vi "VCO-sctl-3.vi"(6 "Ready For Output":bool, 8 "Input Valid":bool, 10 "param":T1={"base freq (Hz)"=[20123.0, 20123.0, 20123.0], "P gain"=[1234.0, 1234.0, 1234.0], "I gain"=[1.0, 1.0, 1.0], "LP1 coeffs"=[-1025014616, 2098093632, 165702, -1053286467, 2126356551, 167935, -1025014616, 2098093632, 165702, -1053286467, 2126356551, 167935, -1025014616, 2098093632, 165702, -1053286467, 2126356551, 167935], "scope on"=FALSE, "scope channel"=0, "scope signal"=0, "notch coeff"=[-1025014616, 2098093632, 165702, -1053286467, 2126356551, 167935, -1025014616, 2098093632, 165702]}, 11 "freq error":fxp<+/-,21,11>) -> (0 "Output Valid":bool, 3 "phase":fxp<+,26,1>, 4 "Ready For Input":bool=TRUE)   [LabVIEW 2018, in "SCTL.lvlib"]
doc: "This VI is used in four wire handshake."
uses:
  SCTL.lvlib
  param-sctl-pll.ctl
  <vilib>/rvi/FXPMathLib/FxpAdd/XNode/nifxpmath_Add.xnode
  <vilib>/rvi/FXPMathLib/FxpMul/XNode/nifxpmath_Multiplier.xnode
  <vilib>/rvi/FXPMathLib/sim/FxpSim.dll
panel:
  # "Inputs"
  # "Outputs"
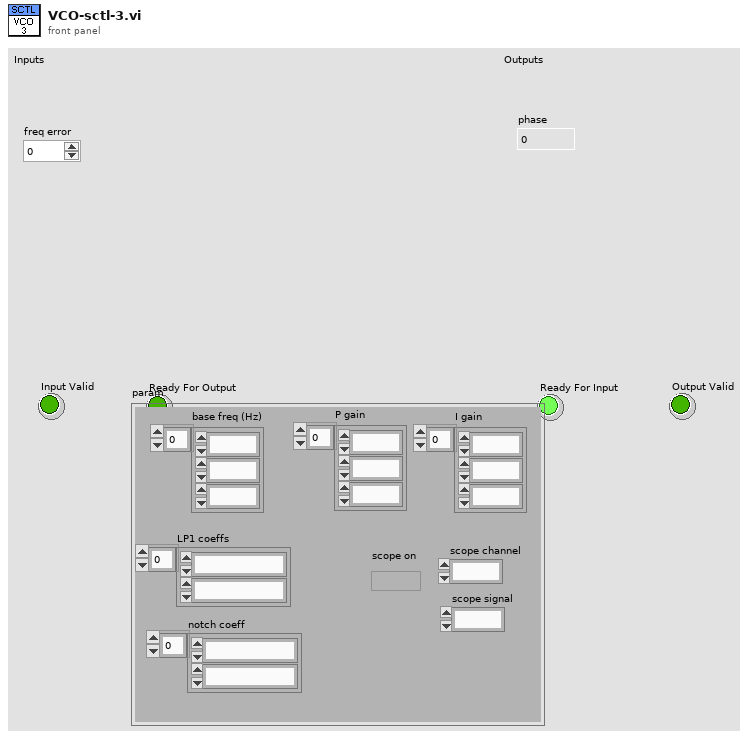
[diagram p1: front panel]
types:
  T1 = typedef "SCTL.lvlib/param-sctl-pll.ctl" = cluster{"base freq (Hz)":fxp<+,17,17>[], "P gain":fxp<+,14,14>[], "I gain":fxp<+,20,6>[], "LP1 coeffs":i32[], "scope on":bool, "scope channel":u8, "scope signal":u8, "notch coeff":i32[]}
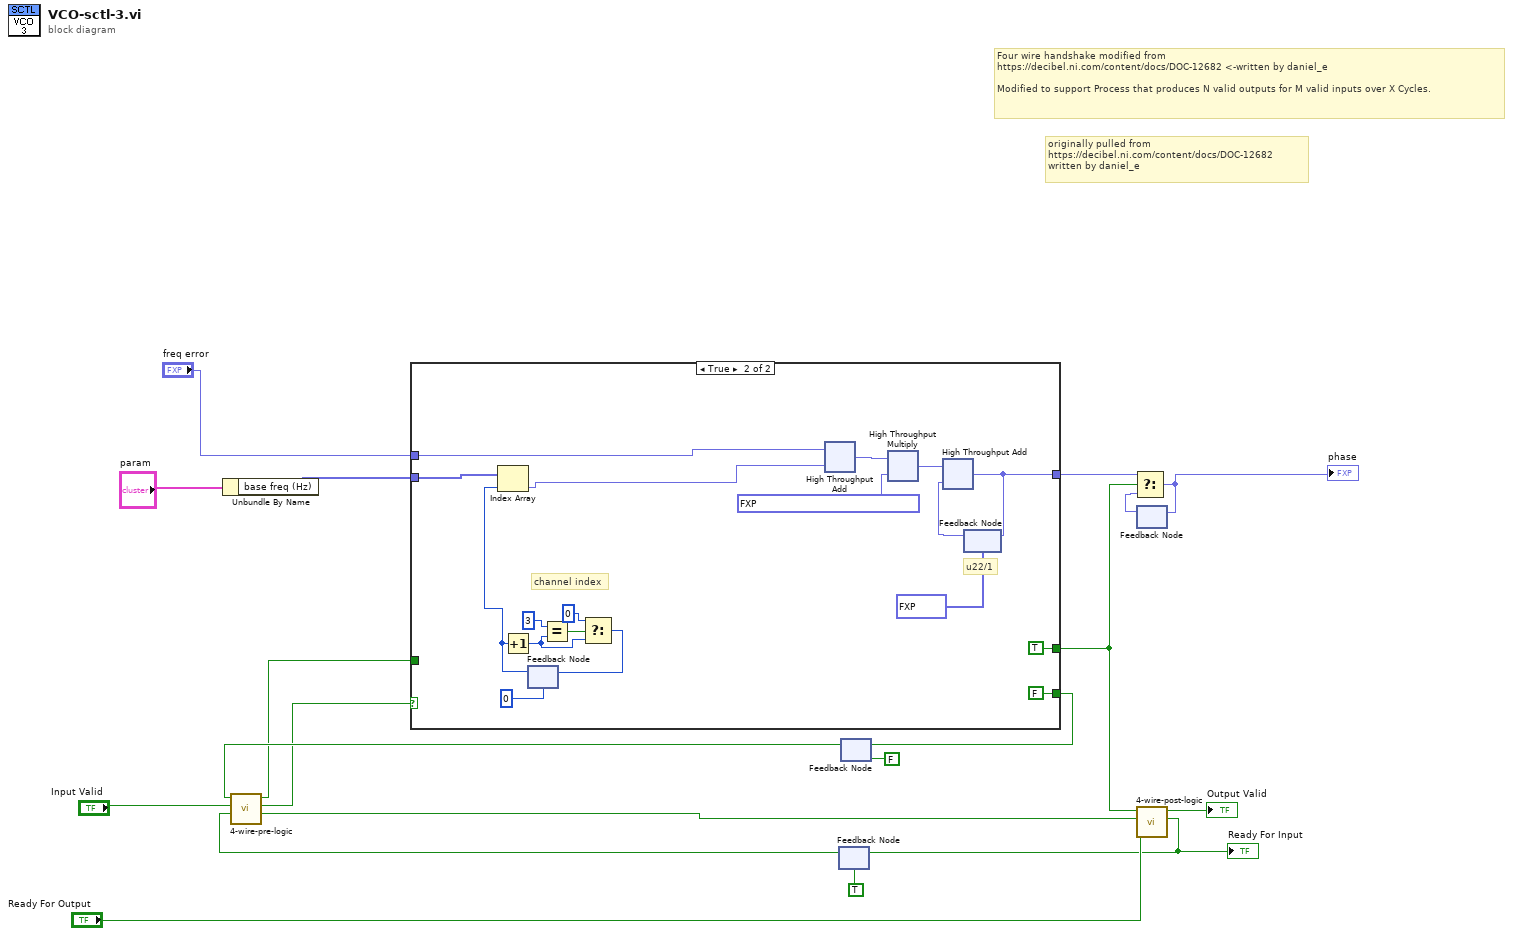
[diagram p0: block diagram]
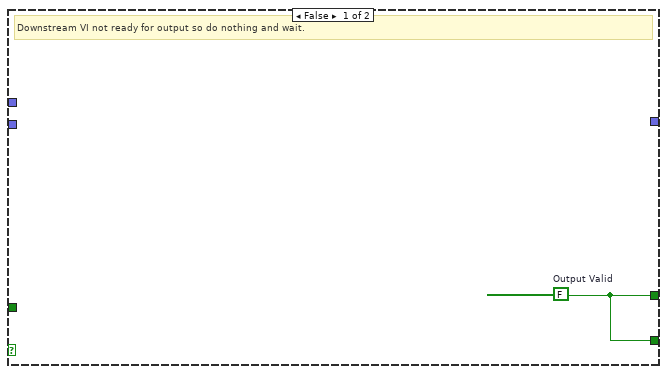
[diagram p2: hidden frame]
diagram:
  # "originally pulled from \nhttps://decibel.ni.com/content/docs/DOC-12682\nwritten by daniel_e"
  # "Four wire handshake modified from \nhttps://decibel.ni.com/content/docs/DOC-12682 <-written by daniel_e\n\nModified to support Process that produces N valid outputs for M valid inputs over X Cycles."
  n1 = Unbundle By Name("param") -> ("base freq (Hz)"=w1:fxp<+,17,17>[])
  n2 = feedback #1(TRUE ("x .and. y?")) -> (w15:bool)
  n3 = feedback #2(FALSE ("x .and. y?")) -> (w13:bool)
  n4 = call "4-wire-pre-logic.vi"("ready for input in"=w15, "Input Valid in"="Input Valid", "needs more iter in"=w13) -> ("register state out"=w18:bool, "excecute"=w12:bool, "buffer input!"=w4:bool)  [unwired: 6 in]
  n5 = case shown="True" w12 {
    tunnel: [w20 TRUE ("Output Valid")] -> w17
    tunnel: w4 -> [_ _]
    tunnel: [w20 FALSE ("Output Valid")] -> w11
    tunnel: "freq error" -> [_ w22]
    tunnel: [_ w33] -> w6
    tunnel: w1 -> [_ w25]
    frame False {
      w20 = FALSE  # Output Valid
      # "Downstream VI not ready for output so do nothing and wait."
    }
    frame True {
      # "channel index"
      # "u22/1"
      n6 = feedback #3(i16 0) -> (w24:i16)
      n7 = Index Array(array=w25, index=w24) -> (element=w21:fxp<+,17,17>)
      n8 = Increment(x=w24) -> (x+1=w26:i16)
      n9 = Equal?(x=i16 3, y=w26) -> (x = y?=w31:bool)
      n10 = Select(t=i16 0, s=w31, f=w26) -> (s? t:f=w28:i16)
      n11 = feedback-in #3(w28) -> ()
      n12 = xnode ("High Throughput Add")("x"=w22, "y"=w21) -> ("x+y"=w34:fxp<+,27,17>)
      n13 = xnode ("High Throughput Multiply")("x"=w34, "y"=fxp<+,14,-18> 2.00001522898674e-06) -> ("x*y"=w36:fxp<+,26,1>)
      n14 = feedback #4(fxp<+,26,1>[] [0.0, 0.0, 0.0]) -> (w35:fxp<+,26,1>)
      n15 = xnode ("High Throughput Add")("x"=w36, "y"=w35) -> ("x+y"=w33:fxp<+,26,1>)
      n16 = feedback-in #4(w33) -> ()
    }
  }
  n17 = feedback-in #2(w11) -> ()
  n18 = feedback #5() -> (w3:fxp<+,26,1>)  [unwired: 1 in]
  n19 = Select(t=w6, s=w17, f=w3) -> (s? t:f=w16:fxp<+,26,1>)
  "phase" <- w16
  n20 = feedback-in #5(w16) -> ()
  n21 = call "4-wire-post-logic.vi"("Ready For Output in"="Ready For Output", "register state in"=w18, "output valid in"=w17) -> ("ready for input out"=w8:bool, "output valid out"=→"Output Valid":bool)  [unwired: 7 in]
  "Ready For Input" <- w8
  n22 = feedback-in #1(w8) -> ()
